vi "VirtualEditInterface.vi"(8 "error in (no error)":errorcluster, 11 "Project.lvclass In":refnum<class "Project.lvclass">) -> (0 "error out":errorcluster, 3 "Project.lvclass Out":refnum<class "Project.lvclass">)   [LabVIEW 2014, in "Project.lvclass"]
uses:
  Project.lvclass
  Virtual/Control/AllVirtualTypeData.ctl
  Controls/Mode Controls.ctl
  Singleton.lvclass/Singleton.lvclass/Singleton.ctl
  SystemData.lvclass/SystemData.lvclass/SystemData.ctl
  Singleton.lvclass/ReadDataVariant.vi
  Singleton.lvclass/WriteDataVariant.vi
  Singleton.lvclass/Constructor.vi
  Message Queue/Enqueue Message (Single).vi
  SystemData.lvclass/SystemData.lvclass
  StepData/StepData.lvclass
  Virtual/VirtualOrigin.lvclass
  Message Queue/Message Queue.lvlib
panel:
  in  "RVS":bool caption="Add"
  in  "FWD":bool caption="Add"
  in  "Axis":u16(ring)=1 items=["X"=1, "Y"=2, "Z"=3, "Rotation"=4]
  in  "SearchSetting":T1={"Search Name"="", "Start X"=0.0, "Increase X"=0.0, "X Step"=1, "Start Y"=0.0, "Increase Y"=0.0, "Y Step"=1, "Sensor"=0} {"Y Step" min=1 step=1; "X Step" min=1 step=1}
  in  "Delete":bool
  in  "Modify":bool
  in  "Add":bool
  in  "SearchList":i32(listbox)
  in  "ProjectList":i32(listbox)
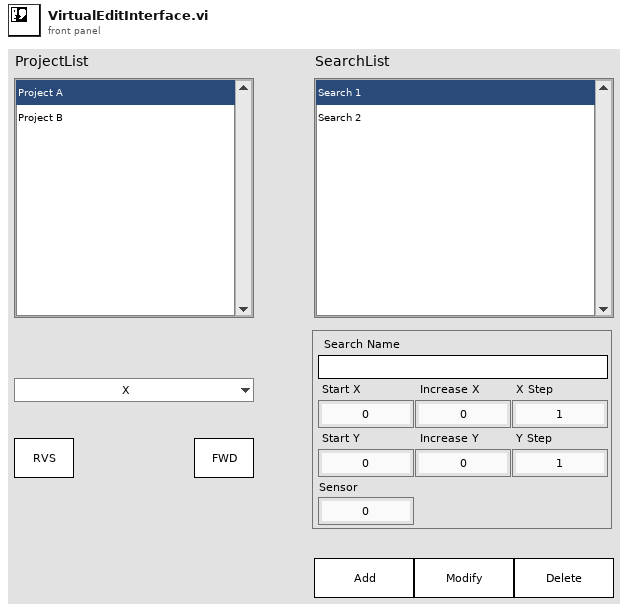
[diagram p1: front panel]
types:
  T1 = typedef "VirtualOrigin.lvclass/AllVirtualTypeData.ctl" = cluster{"Search Name":string, "Start X":dbl, "Increase X":dbl, "X Step":i32, "Start Y":dbl, "Increase Y":dbl, "Y Step":i32, "Sensor":i32}
  T2 = typedef "Mode Controls.ctl" = enum16{"Auto", "Virtual", "Home", "Standby"}
  T3 = typedef "SystemData.lvclass/SystemDataTypeDefine.ctl" = cluster{"Message":T4, "ThisVIParameter":cluster{"Stop":refnum<user-event>, "VI Path":path, "Data Path":path, "This VI Ref":refnum<vi>, "UI Ctrls":T5}, "DBLink":string, "DeployProject":string, "Project.lvclass":refnum<class "Project.lvclass">, "StepDataArray":refnum<class "StepData.lvclass">[], "RuntimeIdx":i32, "HomeIdx":i32, "DAQ Hardware":T6, "Serial Settings":cluster{"VISA":refnum<visa-resource-name>, "Baud Rate":u32, "Data Bits":u16, "Parity":enum16{"None", "Odd", "Even", "Mark", "Space"}, "Stop Bits":u16, "Flow Control":u16}, "Display":T7, "Streaming":T8, "Read":T9, "VirtualDataArray":refnum<class "VirtualOrigin.lvclass">[], "VirtualIdx":i32, "VirtualXIdx":i32, "VirtualYIdx":i32, "VirtualXArray":dbl[], "VirtualYArray":dbl[], "Mode":T2, "Standby":dbl[], "StandbyIdx":i32}
  T4 = typedef "Message Queue.lvlib/All Message Queues.ctl" = cluster{"UI":refnum<queue>, "Task":refnum<queue>, "Motor":refnum<queue>, "DAQ":refnum<queue>, "Logging":refnum<queue>}
  T5 = typedef "UI Controls.ctl" = cluster{"Menu":refnum<k9>, "Start":refnum<vi>, "Stop":refnum<vi>, "Home":refnum<vi>, "Virtual":refnum<vi>, "Save":refnum<vi>}
  T6 = typedef "NIDAQ.lvlib/DAQHardware.ctl" = cluster{"Task":refnum<k21>, "Max":dbl, "min":dbl, "Samples Rate":dbl, "Channels":tag[]}
  T7 = typedef "All Display Notifiers.ctl" = cluster{"DataArray":refnum<queue>, "X":refnum<queue>, "Y":refnum<queue>, "Z":refnum<queue>, "R":refnum<queue>, "Data":refnum<queue>}
  T8 = typedef "Streaming.ctl" = cluster{"Datas":refnum<queue>, "Ready X":dbl, "Ready Y":dbl, "Ready Z":dbl, "Ready R":dbl, "DataArray":dbl[][]}
  T9 = typedef "StepData.lvclass/MeasureData.ctl" = cluster{"Sensor No.":i32, "Log?":bool}
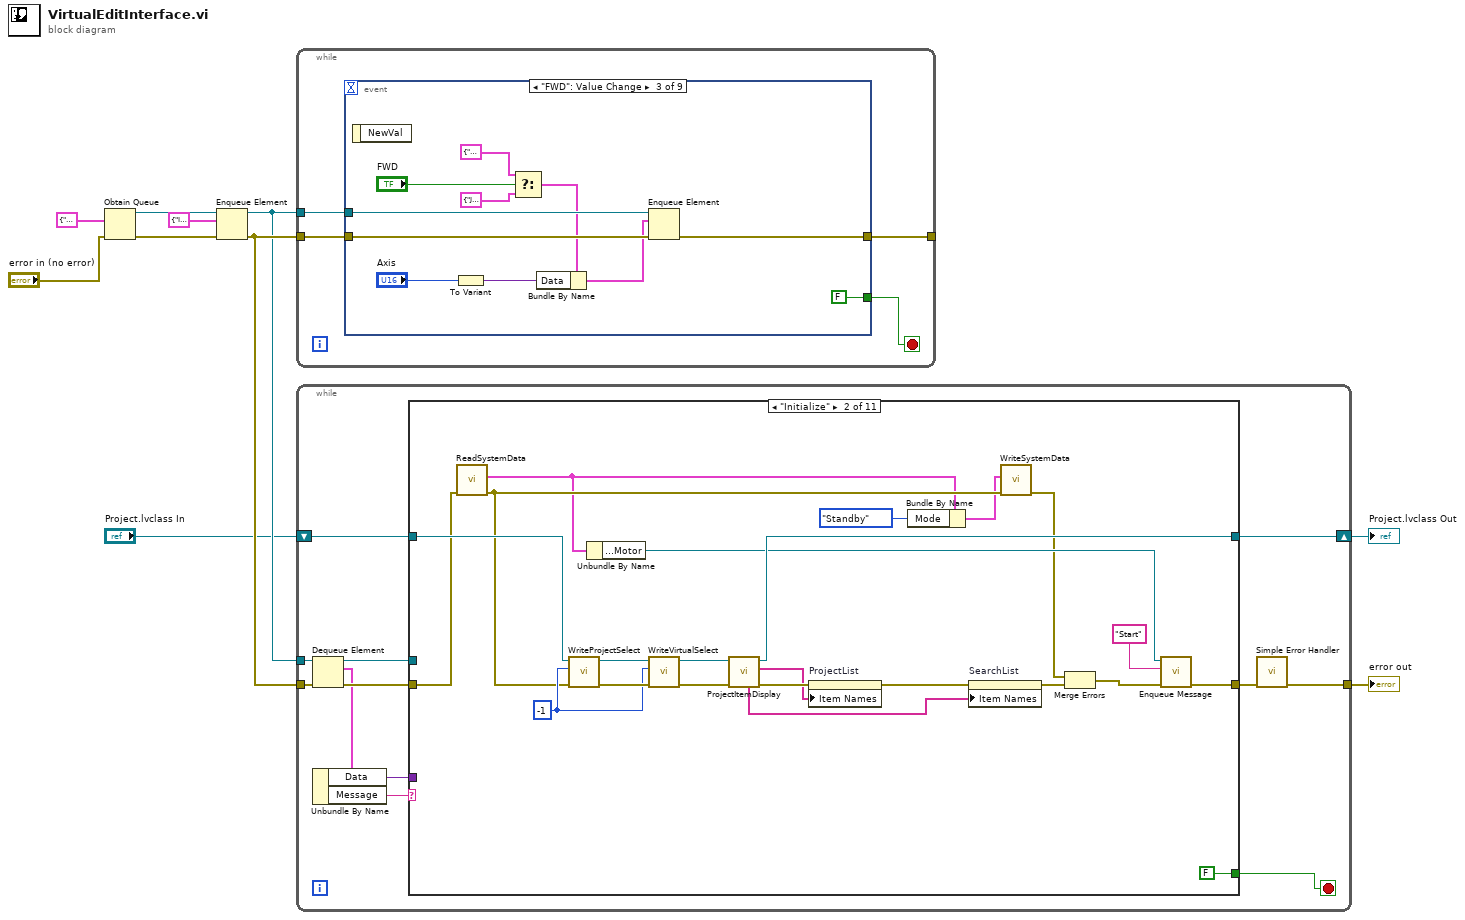
[diagram p0: block diagram]
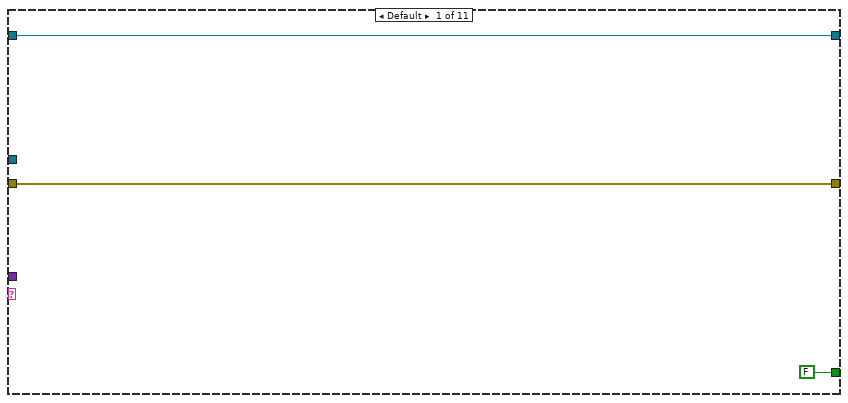
[diagram p2: hidden frame]
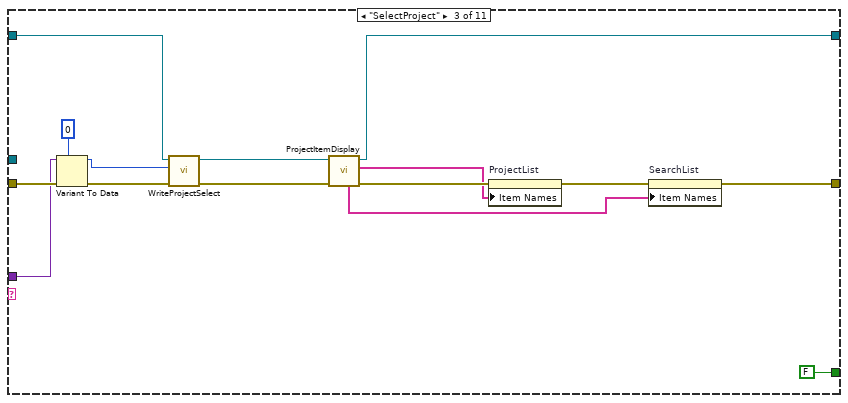
[diagram p3: hidden frame]
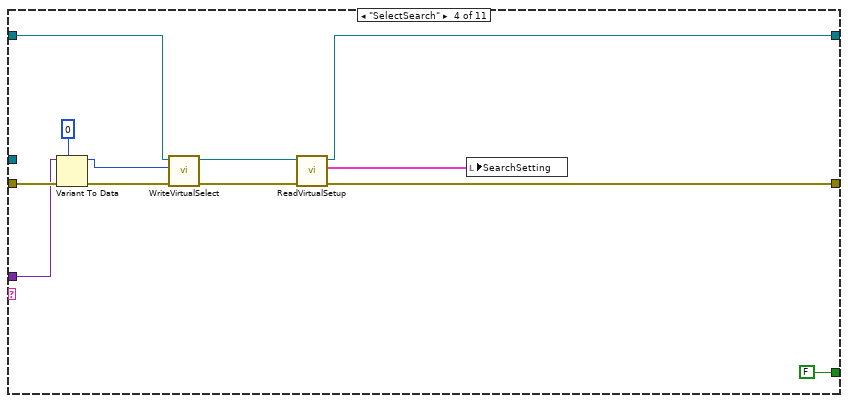
[diagram p4: hidden frame]
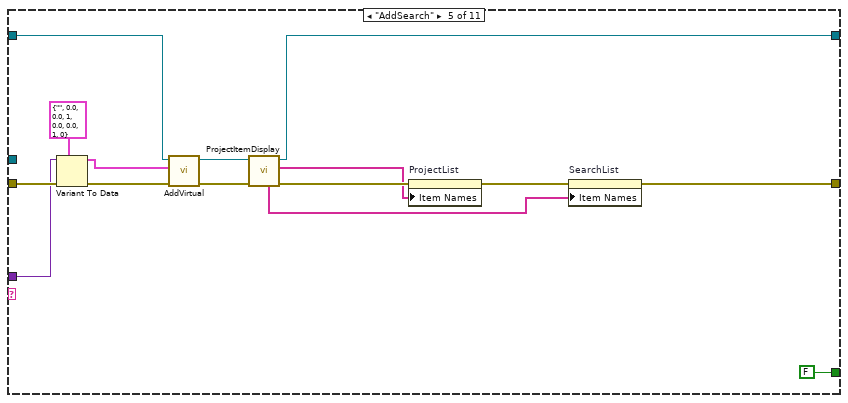
[diagram p5: hidden frame]
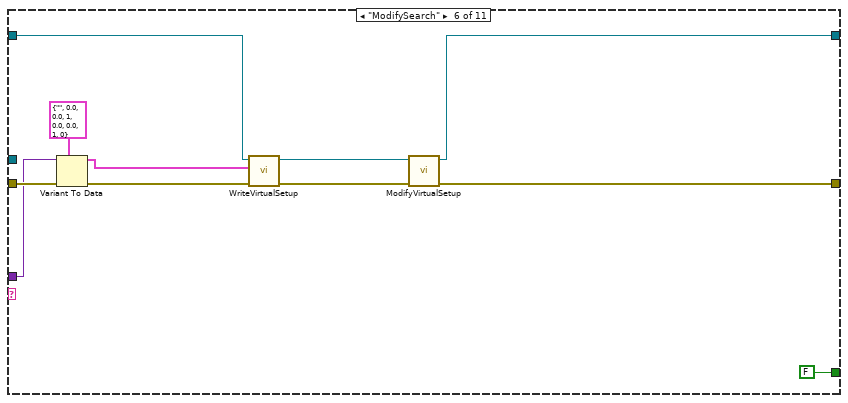
[diagram p6: hidden frame]
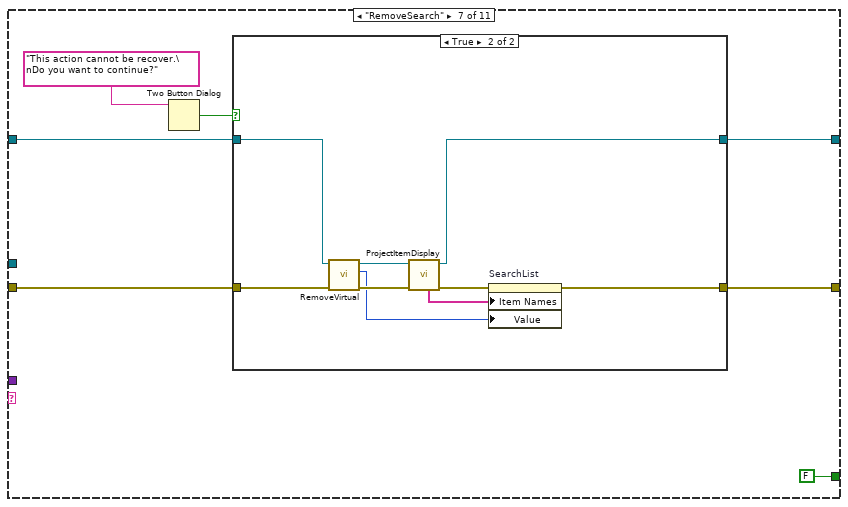
[diagram p7: hidden frame]
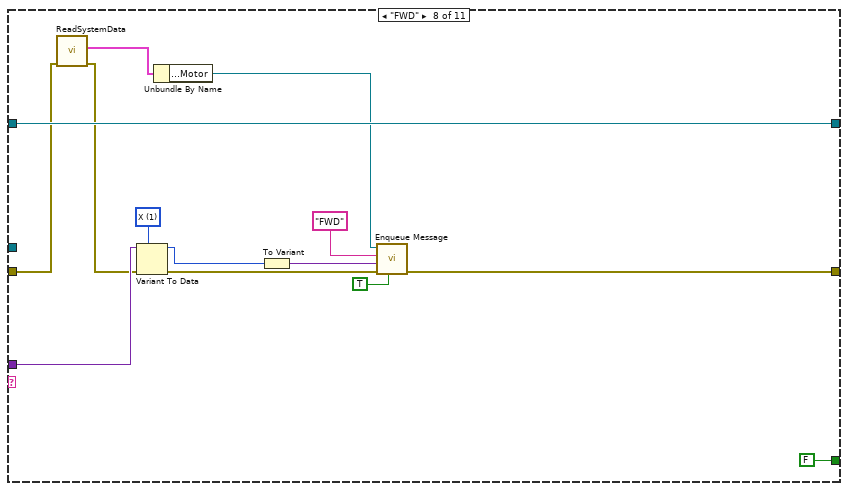
[diagram p9: hidden frame]
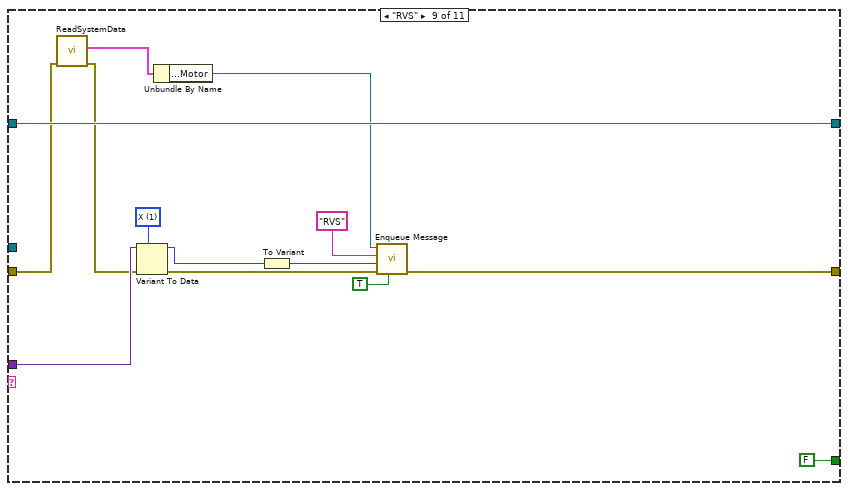
[diagram p10: hidden frame]
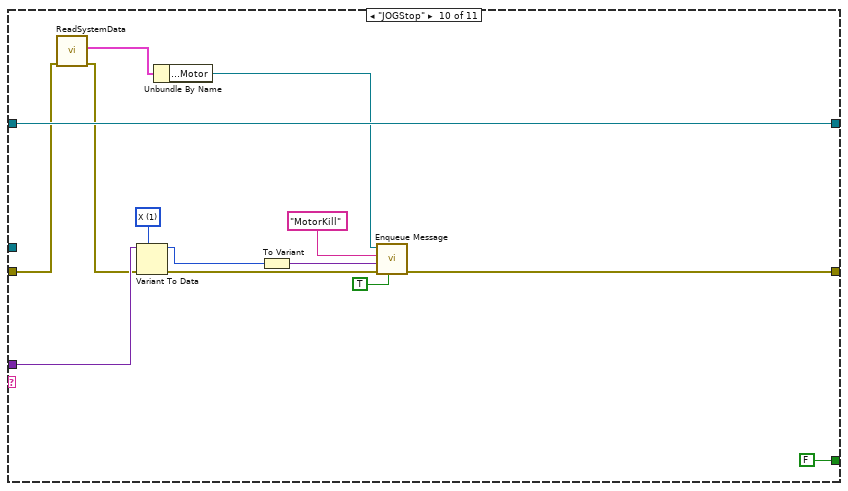
[diagram p11: hidden frame]
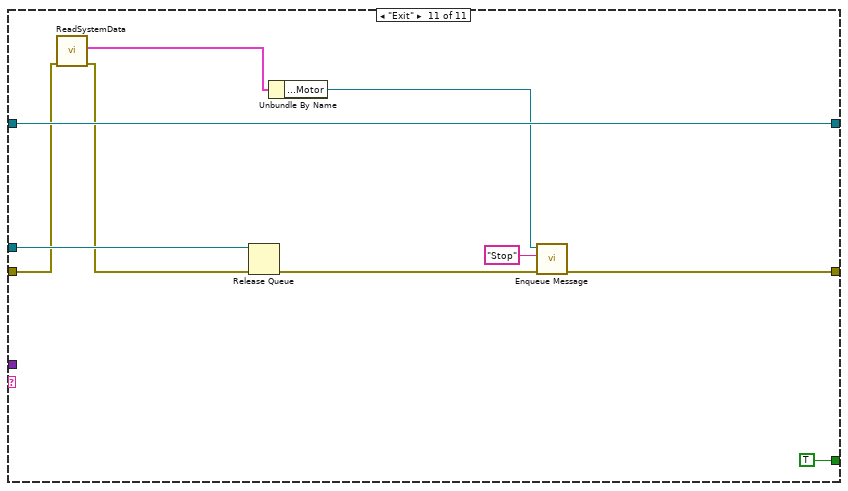
[diagram p12: hidden frame]
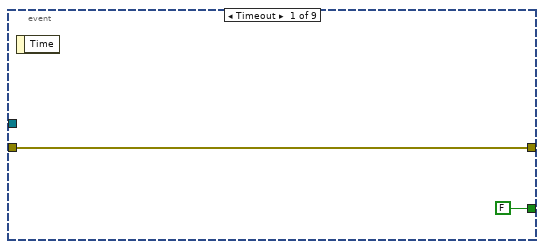
[diagram p13: hidden frame]
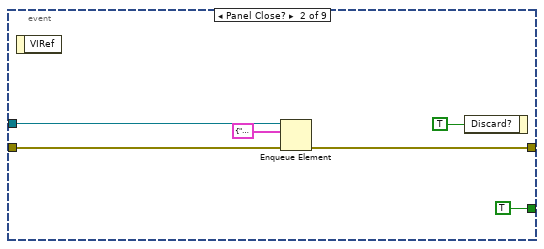
[diagram p14: hidden frame]
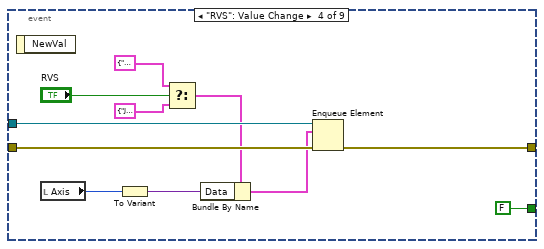
[diagram p15: hidden frame]
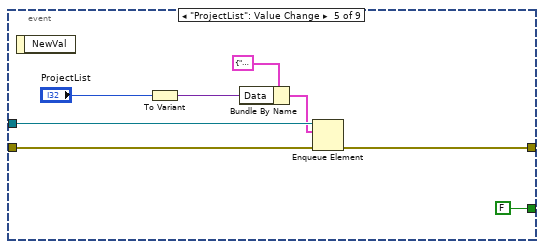
[diagram p16: hidden frame]
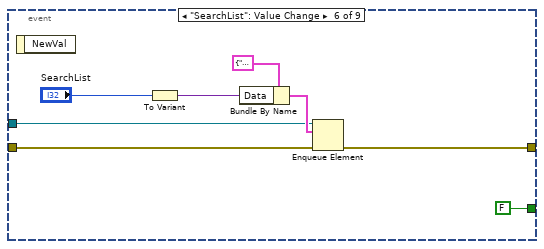
[diagram p17: hidden frame]
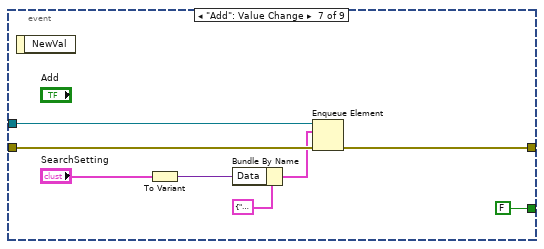
[diagram p18: hidden frame]
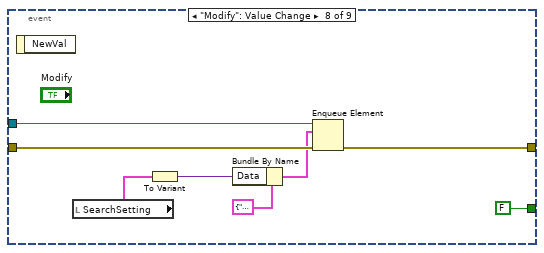
[diagram p19: hidden frame]
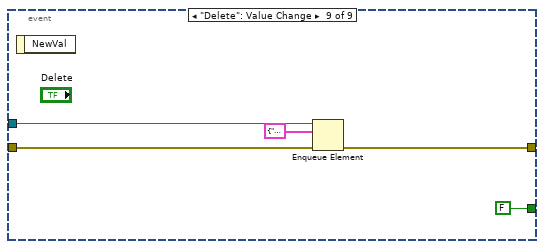
[diagram p20: hidden frame]
diagram:
  n1 = Obtain Queue(element data type=cluster{"Message":string, "Data":variant} {"Message"="", "Data"=variant}, error in (no error)="error in (no error)") -> (queue out=w9:refnum<queue>, error out=w8:errorcluster)  [unwired: 3 in, 1 out]
  n2 = Enqueue Element(queue=w9, element=cluster{"Message":string, "Data":variant} {"Message"="Initialize", "Data"=variant}, error in (no error)=w8) -> (queue out=w6:refnum<queue>, error out=w7:errorcluster)  [unwired: 1 in, 1 out]
  n3 = while {
    tunnel: w6 -> [w13]
    tunnel: w7 -> [w12]
    tunnel: [w11] -> _
    stop <- w14 stop-if-true
    n4 = event shown="[2] \"FWD\": Value Change" {
      selector: _ -> [_ _ _ _ _ _ _ _ _]
      dyn-events: _ -> [_ _ _ _ _ _ _ _ _]
      timeout: _ -> [_ _ _ _ _ _ _ _ _]
      tunnel: [FALSE ("Discard?") TRUE ("Discard?") FALSE ("Discard?") FALSE ("Discard?") FALSE ("Discard?") FALSE ("Discard?") FALSE ("Discard?") FALSE ("Discard?") FALSE ("Discard?")] -> w14
      tunnel: w13 -> [_ w21 w33 w44 w52 w56 w67 w75 w80]
      tunnel: w12 -> [w15 w20 w32 w43 w51 w55 w66 w74 w79]
      tunnel: [w15 w17 w23 w34 w45 w53 w61 w69 w77] -> w11
      event Timeout {
        n5 = event-data() -> ()  [unwired: 1 in, 1 out]
      }
      event Panel Close? {
        n6 = event-data() -> ()  [unwired: 1 in, 1 out]
        n7 = Enqueue Element(queue=w21, element=cluster{"Message":string, "Data":variant} {"Message"="Exit", "Data"=variant}, error in (no error)=w20) -> (error out=w17:errorcluster)  [unwired: 1 in, 2 out]
        n8 = event-data("Discard?"=TRUE) -> ()  [unwired: 1 in, 1 out]
      }
      event "FWD": Value Change {
        n9 = event-data() -> ()  [unwired: 1 in, 1 out]
        n10 = To Variant(anything="Axis") -> (Variant=w29:variant)
        n11 = Select(t=cluster{"Message":string, "Data":variant} {"Message"="FWD", "Data"=variant} ("element"), s="FWD", f=cluster{"Message":string, "Data":variant} {"Message"="JOGStop", "Data"=variant} ("element")) -> (s? t:f=w25:cluster{"Message":string, "Data":variant})
        n12 = Bundle By Name(cluster=w25, "Data"=w29) -> (w30:cluster{"Message":string, "Data":variant})
        n13 = Enqueue Element(queue=w33, element=w30, error in (no error)=w32) -> (error out=w23:errorcluster)  [unwired: 1 in, 2 out]
      }
      event "RVS": Value Change {
        n14 = event-data() -> ()  [unwired: 1 in, 1 out]
        n15 = local read "Axis"() -> (w40:u16)
        n16 = To Variant(anything=w40) -> (Variant=w41:variant)
        n17 = Select(t=cluster{"Message":string, "Data":variant} {"Message"="RVS", "Data"=variant} ("element"), s="RVS", f=cluster{"Message":string, "Data":variant} {"Message"="JOGStop", "Data"=variant} ("element")) -> (s? t:f=w36:cluster{"Message":string, "Data":variant})
        n18 = Bundle By Name(cluster=w36, "Data"=w41) -> (w42:cluster{"Message":string, "Data":variant})
        n19 = Enqueue Element(queue=w44, element=w42, error in (no error)=w43) -> (error out=w34:errorcluster)  [unwired: 1 in, 2 out]
      }
      event "ProjectList": Value Change {
        n20 = event-data() -> ()  [unwired: 1 in, 1 out]
        n21 = To Variant(anything="ProjectList") -> (Variant=w47:variant)
        n22 = Bundle By Name(cluster=cluster{"Message":string, "Data":variant} {"Message"="SelectProject", "Data"=variant} ("element"), "Data"=w47) -> (w46:cluster{"Message":string, "Data":variant})
        n23 = Enqueue Element(queue=w52, element=w46, error in (no error)=w51) -> (error out=w45:errorcluster)  [unwired: 1 in, 2 out]
      }
      event "SearchList": Value Change {
        n24 = event-data() -> ()  [unwired: 1 in, 1 out]
        n25 = To Variant(anything="SearchList") -> (Variant=w57:variant)
        n26 = Bundle By Name(cluster=cluster{"Message":string, "Data":variant} {"Message"="SelectSearch", "Data"=variant} ("element"), "Data"=w57) -> (w59:cluster{"Message":string, "Data":variant})
        n27 = Enqueue Element(queue=w56, element=w59, error in (no error)=w55) -> (error out=w53:errorcluster)  [unwired: 1 in, 2 out]
      }
      event "Add": Value Change {
        n28 = event-data() -> ()  [unwired: 1 in, 1 out]
        n29 = To Variant(anything="SearchSetting") -> (Variant=w64:variant)
        n30 = Bundle By Name(cluster=cluster{"Message":string, "Data":variant} {"Message"="AddSearch", "Data"=variant} ("element"), "Data"=w64) -> (w62:cluster{"Message":string, "Data":variant})
        n31 = Enqueue Element(queue=w67, element=w62, error in (no error)=w66) -> (error out=w61:errorcluster)  [unwired: 1 in, 2 out]
      }
      event "Modify": Value Change {
        n32 = event-data() -> ()  [unwired: 1 in, 1 out]
        n33 = local read "SearchSetting"() -> (w70:T1)
        n34 = To Variant(anything=w70) -> (Variant=w71:variant)
        n35 = Bundle By Name(cluster=cluster{"Message":string, "Data":variant} {"Message"="ModifySearch", "Data"=variant} ("element"), "Data"=w71) -> (w72:cluster{"Message":string, "Data":variant})
        n36 = Enqueue Element(queue=w75, element=w72, error in (no error)=w74) -> (error out=w69:errorcluster)  [unwired: 1 in, 2 out]
      }
      event "Delete": Value Change {
        n37 = event-data() -> ()  [unwired: 1 in, 1 out]
        n38 = Enqueue Element(queue=w80, element=cluster{"Message":string, "Data":variant} {"Message"="RemoveSearch", "Data"=variant}, error in (no error)=w79) -> (error out=w77:errorcluster)  [unwired: 1 in, 2 out]
      }
    }
  }
  n39 = while {
    tunnel: w7 -> [w93]
    tunnel: w6 -> [w92]
    shift-right: [w85] -> w3
    shift-left: "Project.lvclass In" -> [w86]
    tunnel: [w83] -> w1
    stop <- w82 stop-if-true
    n40 = Dequeue Element(queue=w92, error in (no error)=w93) -> (queue out=w87:refnum<queue>, element=w90:cluster{"Message":string, "Data":variant}, error out=w91:errorcluster)  [unwired: 1 in, 1 out]
    n41 = Unbundle By Name(w90) -> ("Data"=w88:variant, "Message"=w89:string)
    n42 = case shown="\"Initialize\"" w89 {
      tunnel: w91 -> [w94 w107 w133 w145 w160 w170 w175 w201 w215 w229 w239]
      tunnel: w88 -> [_ _ w125 w143 w159 w169 _ w203 w217 w231 _]
      tunnel: [FALSE FALSE FALSE FALSE FALSE FALSE FALSE FALSE FALSE FALSE TRUE] -> w82
      tunnel: w87 -> [_ _ _ _ _ _ _ _ _ _ w242]
      tunnel: w86 -> [w95 w118 w129 w140 w157 w167 w177 w204 w218 w232 w240]
      tunnel: [w95 w112 w126 w137 w152 w171 w176 w204 w218 w232 w240] -> w85
      tunnel: [w94 w103 w120 w135 w147 w162 w173 w193 w207 w221 w234] -> w84
      frame Default {
      }
      frame "Initialize" {
        w115 = -1 ("ProjectSelectIdx")
        n43 = call "ReadSystemData.vi"("error in (no error)"=w107) -> ("error out"=w106:errorcluster, "SystemData Out"=w102:T3)  [unwired: 9 in]
        n44 = call "WriteProjectSelect.vi"("error in (no error)"=w106, "ProjectSelectIdx"=w115, "Project.lvclass In"=w118) -> ("error out"=w116:errorcluster, "Project.lvclass Out"=w117:refnum<class "Project.lvclass">)  [unwired: 7 in]
        n45 = Unbundle By Name(w102) -> ("Message.Motor"=w101:refnum<queue>)
        n46 = call "WriteVirtualSelect.vi"("error in (no error)"=w116, "VirtualSelectIdx"=w115, "Project.lvclass In"=w117) -> ("error out"=w113:errorcluster, "Project.lvclass Out"=w114:refnum<class "Project.lvclass">)  [unwired: 7 in]
        n47 = call "ProjectItemDisplay.vi"("error in (no error)"=w113, "Project.lvclass In"=w114) -> ("error out"=w111:errorcluster, "ProjectNames"=w109:string[], "Project.lvclass Out"=w112:refnum<class "Project.lvclass">, "VirtualNames"=w108:string[])  [unwired: 5 in, 1 out]
        n48 = property on="ProjectList" class="LstBox (strict)"(error in=w111, "Item Names"=w109) -> (error out=w110:errorcluster)  [unwired: 1 in, 1 out]
        n49 = Bundle By Name(cluster=w102, "Mode"=Mode_Controls."Standby") -> (w104:T3)
        n50 = property on="SearchList" class="LstBox (strict)"(error in=w110, "Item Names"=w108) -> (error out=w100:errorcluster)  [unwired: 1 in, 1 out]
        n51 = call "WriteSystemData.vi"("error in (no error)"=w106, "SystemData In"=w104) -> ("error out"=w98:errorcluster)  [unwired: 9 in]
        n52 = Merge Errors(w98, w100) -> (w99:errorcluster)
        n53 = call-poly "Enqueue Message.vi"("error in (no error)"=w99, "Message"="Start", "Message Queue"=w101) -> ("error out"=w103:errorcluster)  [unwired: 7 in, 1 out]
      }
      frame "SelectProject" {
        n54 = Variant To Data(error in=w133, type=0, Variant=w125) -> (data=w130:i32, error out=w131:errorcluster)
        n55 = call "WriteProjectSelect.vi"("error in (no error)"=w131, "ProjectSelectIdx"=w130, "Project.lvclass In"=w129) -> ("error out"=w128:errorcluster, "Project.lvclass Out"=w127:refnum<class "Project.lvclass">)  [unwired: 7 in]
        n56 = call "ProjectItemDisplay.vi"("error in (no error)"=w128, "Project.lvclass In"=w127) -> ("error out"=w124:errorcluster, "ProjectNames"=w123:string[], "Project.lvclass Out"=w126:refnum<class "Project.lvclass">, "VirtualNames"=w121:string[])  [unwired: 5 in, 1 out]
        n57 = property on="ProjectList" class="LstBox (strict)"(error in=w124, "Item Names"=w123) -> (error out=w122:errorcluster)  [unwired: 1 in, 1 out]
        n58 = property on="SearchList" class="LstBox (strict)"(error in=w122, "Item Names"=w121) -> (error out=w120:errorcluster)  [unwired: 1 in, 1 out]
      }
      frame "SelectSearch" {
        n59 = Variant To Data(error in=w145, type=0, Variant=w143) -> (data=w141:i32, error out=w142:errorcluster)
        n60 = call "WriteVirtualSelect.vi"("error in (no error)"=w142, "VirtualSelectIdx"=w141, "Project.lvclass In"=w140) -> ("error out"=w139:errorcluster, "Project.lvclass Out"=w138:refnum<class "Project.lvclass">)  [unwired: 7 in]
        n61 = call "ReadVirtualSetup.vi"("error in (no error)"=w139, "Project.lvclass In"=w138) -> ("error out"=w135:errorcluster, "VirtualTypeData"=w136:T1, "Project.lvclass Out"=w137:refnum<class "Project.lvclass">)  [unwired: 7 in]
        n62 = local write "SearchSetting"(w136) -> ()
      }
      frame "AddSearch" {
        n63 = Variant To Data(error in=w160, type=T1 {"Search Name"="", "Start X"=0.0, "Increase X"=0.0, "X Step"=1, "Start Y"=0.0, "Increase Y"=0.0, "Y Step"=1, "Sensor"=0} ("SearchSetting"), Variant=w159) -> (data=w156:T1, error out=w155:errorcluster)
        n64 = call "AddVirtual.vi"("error in (no error)"=w155, "AllVirtualTypeData"=w156, "Project.lvclass In"=w157) -> ("error out"=w153:errorcluster, "Project.lvclass Out"=w154:refnum<class "Project.lvclass">)  [unwired: 7 in]
        n65 = call "ProjectItemDisplay.vi"("error in (no error)"=w153, "Project.lvclass In"=w154) -> ("error out"=w151:errorcluster, "ProjectNames"=w150:string[], "Project.lvclass Out"=w152:refnum<class "Project.lvclass">, "VirtualNames"=w148:string[])  [unwired: 5 in, 1 out]
        n66 = property on="ProjectList" class="LstBox (strict)"(error in=w151, "Item Names"=w150) -> (error out=w149:errorcluster)  [unwired: 1 in, 1 out]
        n67 = property on="SearchList" class="LstBox (strict)"(error in=w149, "Item Names"=w148) -> (error out=w147:errorcluster)  [unwired: 1 in, 1 out]
      }
      frame "ModifySearch" {
        n68 = Variant To Data(error in=w170, type=T1 {"Search Name"="", "Start X"=0.0, "Increase X"=0.0, "X Step"=1, "Start Y"=0.0, "Increase Y"=0.0, "Y Step"=1, "Sensor"=0} ("SearchSetting"), Variant=w169) -> (data=w164:T1, error out=w163:errorcluster)
        n69 = call "WriteVirtualSetup.vi"("error in (no error)"=w163, "AllVirtualTypeData"=w164, "Project.lvclass In"=w167) -> ("error out"=w165:errorcluster, "Project.lvclass Out"=w166:refnum<class "Project.lvclass">)  [unwired: 7 in]
        n70 = call "ModifyVirtualSetup.vi"("error in (no error)"=w165, "Project.lvclass In"=w166) -> ("error out"=w162:errorcluster, "Project.lvclass Out"=w171:refnum<class "Project.lvclass">)  [unwired: 8 in]
      }
      frame "RemoveSearch" {
        n71 = Two Button Dialog(message="This action cannot be recover.\nDo you want to continue?") -> (T button?=w178:bool)  [unwired: 2 in]
        n72 = case shown="True" w178 {
          tunnel: w177 -> [w181 w185]
          tunnel: [w181 w184] -> w176
          tunnel: w175 -> [w180 w183]
          tunnel: [w180 w182] -> w173
          frame False {
          }
          frame True {
            n73 = call "RemoveVirtual.vi"("error in (no error)"=w183, "Project.lvclass In"=w185) -> ("error out"=w189:errorcluster, "VirtualIdx"=w186:i32, "Project.lvclass Out"=w190:refnum<class "Project.lvclass">)  [unwired: 7 in]
            n74 = call "ProjectItemDisplay.vi"("error in (no error)"=w189, "Project.lvclass In"=w190) -> ("error out"=w188:errorcluster, "Project.lvclass Out"=w184:refnum<class "Project.lvclass">, "VirtualNames"=w187:string[])  [unwired: 5 in, 2 out]
            n75 = property on="SearchList" class="LstBox (strict)"(error in=w188, "Item Names"=w187, "Value"=w186) -> (error out=w182:errorcluster)  [unwired: 1 in, 1 out]
          }
        }
      }
      frame "FWD" {
        w196 = u16 1 items=["X"=1, "Y"=2, "Z"=3, "Rotation"=4] ("Axis")
        n76 = call "ReadSystemData.vi"("error in (no error)"=w201) -> ("error out"=w200:errorcluster, "SystemData Out"=w199:T3)  [unwired: 9 in]
        n77 = Variant To Data(error in=w200, type=w196, Variant=w203) -> (data=w195:u16, error out=w202:errorcluster)
        n78 = Unbundle By Name(w199) -> ("Message.Motor"=w198:refnum<queue>)
        n79 = To Variant(anything=w195) -> (Variant=w194:variant)
        n80 = call-poly "Enqueue Message.vi"("Priority Message? (F)"=TRUE, "error in (no error)"=w202, "Message Data"=w194, "Message"="FWD", "Message Queue"=w198) -> ("error out"=w193:errorcluster)  [unwired: 5 in, 1 out]
      }
      frame "RVS" {
        w210 = u16 1 items=["X"=1, "Y"=2, "Z"=3, "Rotation"=4] ("Axis")
        n81 = call "ReadSystemData.vi"("error in (no error)"=w215) -> ("error out"=w214:errorcluster, "SystemData Out"=w213:T3)  [unwired: 9 in]
        n82 = Variant To Data(error in=w214, type=w210, Variant=w217) -> (data=w209:u16, error out=w216:errorcluster)
        n83 = Unbundle By Name(w213) -> ("Message.Motor"=w212:refnum<queue>)
        n84 = To Variant(anything=w209) -> (Variant=w208:variant)
        n85 = call-poly "Enqueue Message.vi"("Priority Message? (F)"=TRUE, "error in (no error)"=w216, "Message Data"=w208, "Message"="RVS", "Message Queue"=w212) -> ("error out"=w207:errorcluster)  [unwired: 5 in, 1 out]
      }
      frame "JOGStop" {
        w224 = u16 1 items=["X"=1, "Y"=2, "Z"=3, "Rotation"=4] ("Axis")
        n86 = call "ReadSystemData.vi"("error in (no error)"=w229) -> ("error out"=w228:errorcluster, "SystemData Out"=w227:T3)  [unwired: 9 in]
        n87 = Variant To Data(error in=w228, type=w224, Variant=w231) -> (data=w223:u16, error out=w230:errorcluster)
        n88 = Unbundle By Name(w227) -> ("Message.Motor"=w226:refnum<queue>)
        n89 = To Variant(anything=w223) -> (Variant=w222:variant)
        n90 = call-poly "Enqueue Message.vi"("Priority Message? (F)"=TRUE, "error in (no error)"=w230, "Message Data"=w222, "Message"="MotorKill", "Message Queue"=w226) -> ("error out"=w221:errorcluster)  [unwired: 5 in, 1 out]
      }
      frame "Exit" {
        n91 = call "ReadSystemData.vi"("error in (no error)"=w239) -> ("error out"=w238:errorcluster, "SystemData Out"=w235:T3)  [unwired: 9 in]
        n92 = Release Queue(queue=w242, error in (no error)=w238) -> (error out=w237:errorcluster)  [unwired: 1 in, 2 out]
        n93 = Unbundle By Name(w235) -> ("Message.Motor"=w236:refnum<queue>)
        n94 = call-poly "Enqueue Message.vi"("error in (no error)"=w237, "Message"="Stop", "Message Queue"=w236) -> ("error out"=w234:errorcluster)  [unwired: 7 in, 1 out]
      }
    }
    n95 = call <vilib>:"Simple Error Handler.vi"("error in (no error)"=w84) -> ("error out"=w83:errorcluster)  [unwired: 4 in, 4 out]
  }
  "Project.lvclass Out" <- w3
  "error out" <- w1
